vi "Conductus Send Calibration.vi"() -> ()   [LabVIEW 2024]
doc: "This VI loads a calibration file into the Conductus LTC-20 temperature controller. The file is a line of up to 19 characters of ID info, followed by the temperature information in 2 columns of temperature and resistance (sensor value)\nScott Hannahs, NHMFL-FSU, March 1995"
panel:
  in  "Voltage Bias":i32(ring)=1 items=["10 mV", "3 mV", "1 mV", "320 uV", "100 uV", "32 uV", "10 uV"]
  out "?":i32
  in  "Instrument Address":refnum<visa-resource-name>
  out "# of User Tables loaded":i32
  in  "Sensor Type":i32(ring)=4 items=["2V Diode", "6V Diode", "Platinum - 1 mA", "Platinum - 100µA", "Resistance1.0M "]
  out "Curve Table for Calibration #":string
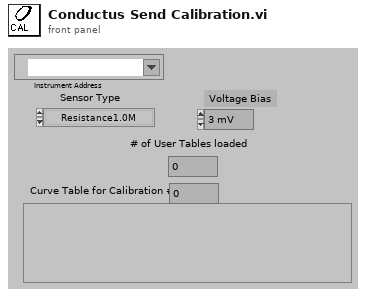
[diagram p1: front panel]
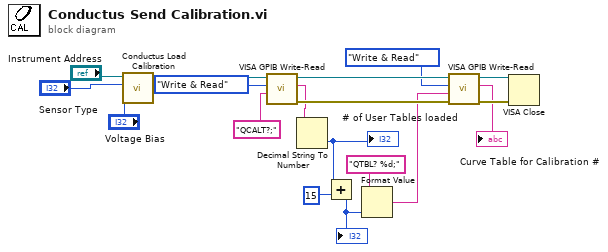
[diagram p0: block diagram]
diagram:
  n1 = call "Conductus Load Calibration.vi"("Voltage Bias"="Voltage Bias", "Sensor Type"="Sensor Type", "Instrument Address"="Instrument Address") -> ("dup VISA session"=w4:refnum<visa-resource-name>)  [unwired: 3 in, 1 out]
  n2 = call "VISA GPIB Write-Read.vi"("Command"="QCALT?;", "Action"=enum16{"Write", "Read", "Write & Read"}."Write & Read", "VISA resource name"=w4) -> ("error out"=w18:errorcluster, "String Returned"=w10:string, "dup VISA Session"=w14:refnum<visa-resource-name>)  [unwired: 5 in, 1 out]
  n3 = Decimal String To Number(string=w10) -> (number=w9:i32)  [unwired: 2 in, 1 out]
  "# of User Tables loaded" <- w9
  n4 = Add(x=w9, y=15) -> (x+y=w11:i32)
  "?" <- w11
  n5 = Format Value(format string="QTBL? %d;", value (0)=w11) -> (output string=w13:string)  [unwired: 1 in]
  n6 = call "VISA GPIB Write-Read.vi"("error in (no error)"=w18, "Command"=w13, "Action"=enum16{"Write", "Read", "Write & Read"}."Write & Read", "VISA resource name"=w14) -> ("error out"=w17:errorcluster, "String Returned"=→"Curve Table for Calibration #":string, "dup VISA Session"=w16:refnum<visa-resource-name>)  [unwired: 4 in, 1 out]
  n7 = VISA Close(VISA resource name=w16, error in (no error)=w17) -> ()  [unwired: 1 out]
